vi "CommandServoPosition.vi"(7 "Debug with FS control?":bool, 8 "Error in":errorcluster, 9 "position [%FS]":dbl(slide) scale=-200.0..200.0, 10 "Suggested Rudder Setpoint":T1 min=-1.0 max=1.0 scale=1.0..-1.0, 11 "PWM Ref In":T2) -> (0 "Error out":errorcluster, 3 "duty cycle [%]":dbl)   [LabVIEW 2013]
doc: "This VI takes in a rudder setpoint in the RudderSuggestedSetpoint typedef (range of -1 to 1) and turns it into a a servo position. It is also passed a zero reference so that the rudder can be reinitialized to a new zero.\n\nAssumptions: there is a bound on the range of the rudder inside of this VI, set in consultation with the ME team. A zero position is also passed into this VI, which then translates an incoming -1 (full port) into the zero position minus half of the bounded range.\n\nThe 'Debug with FS Control?' boolean is made for TestRudderServo.vi, so the user can twiddle the servo around without any 'degrees to servo units' conversion. This should be used with new servos to get the 'degrees to servo units' conversion right.\n\nEric Schneider, March 2014"
uses:
  <vilib>/myRIO/Instrument Drivers/Onboard IO/PWM/typedefs/PWM Reference.ctl
  <vilib>/myRIO/Common/Instrument Driver Framework/Utilities/typedefs/myRIO Generic Hardware Reference.ctl
  <vilib>/myRIO/Common/Instrument Driver Framework/Utilities/typedefs/Hardware Version Enum.ctl
  <vilib>/myRIO/Common/Instrument Driver Framework/Utilities/typedefs/myRIO v1.0 Reference.ctl
  <vilib>/myRIO/Common/Instrument Driver Framework/Utilities/typedefs/Generic FPGA Reference.ctl
  <vilib>/myRIO/Common/Instrument Driver Framework/myRIO v1.0/PWM/typedefs/PWM Channels Enum.ctl
  <vilib>/myRIO/Instrument Drivers/Onboard IO/PWM/typedefs/PWM Configuration.ctl
  Data/TypeDefs/Rudder Set Suggestions.ctl
  <vilib>/Utility/error.llb/Error Cluster From Error Code.vi
  <vilib>/myRIO/Common/Instrument Driver Framework/myRIO v1.0/PWM/vis/myRIO v1.0 Write PWM.vi
  <vilib>/myRIO/Instrument Drivers/Onboard IO/PWM/PWM.lvlib
panel:
  in  "\"Zero\" reference (%FS units)":dbl format="%#_13g"
  in  "%FS per degree":dbl=1.85 format="%#_13g"
  in  "Desired range of rudder (deg)":dbl=60.0 format="%#_13g"
  out "offset [%FS]":dbl
  in  "null offset":bool
  out "pulse width [ms]":dbl=1.5
  in  "freq [Hz]":dbl=50.0
  # "Default settings from MyRIO example servo command code"
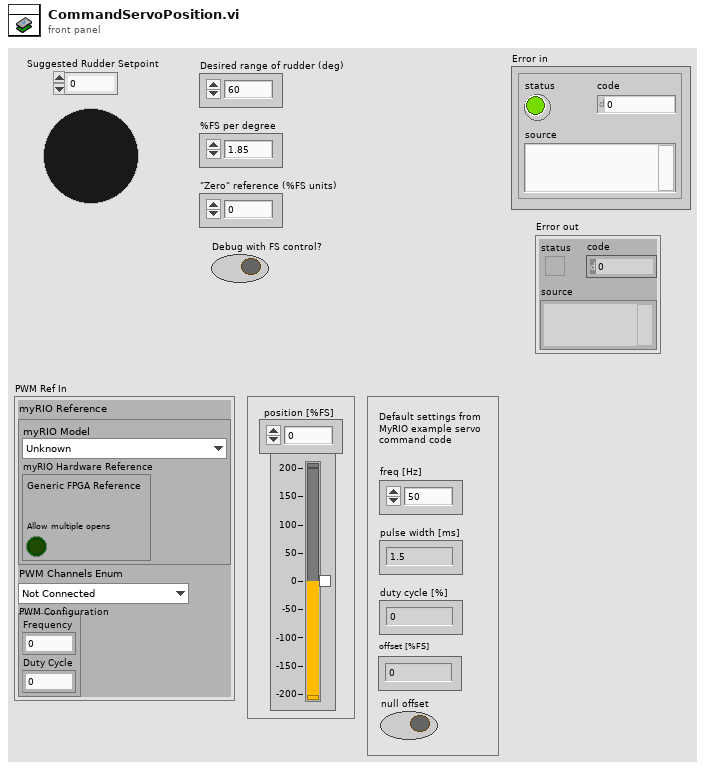
[diagram p1: front panel]
types:
  T1 = typedef "Rudder Set Suggestions.ctl" = dbl
  T2 = typedef "PWM.lvlib/PWM Reference.ctl" = cluster{"myRIO Reference":T3, "PWM Channels Enum":T7, "PWM Configuration":T8}
  T3 = typedef "myRIO Generic Hardware Reference.ctl" = cluster{"myRIO Model":T4, "myRIO Hardware Reference":T5}
  T4 = typedef "Hardware Version Enum.ctl" = enum16{"Unknown", "myRIO-1900", "myRIO-1950"}
  T5 = typedef "myRIO v1.0 Reference.ctl" = cluster{"Generic FPGA Reference":T6, "Allow multiple opens":bool}
  T6 = typedef "Generic FPGA Reference.ctl" = refnum<k20>
  T7 = typedef "PWM Channels Enum.ctl" = enum16{"Not Connected", "C/PWM0", "C/PWM1", "A/PWM0", "A/PWM1", "A/PWM2", "B/PWM0", "B/PWM1", "B/PWM2"}
  T8 = typedef "PWM.lvlib/PWM Configuration.ctl" = cluster{"Frequency":dbl, "Duty Cycle":dbl}
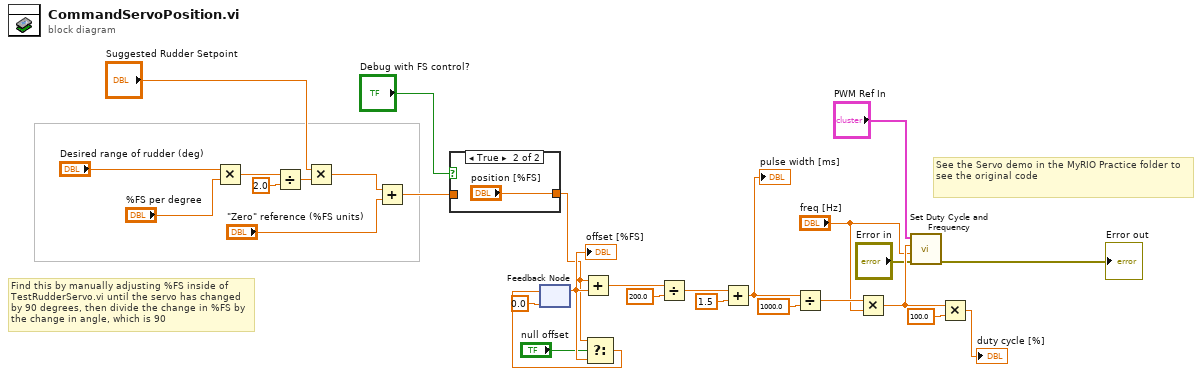
[diagram p0: block diagram]
diagram:
  # "Find this by manually adjusting %FS inside of TestRudderServo.vi until the servo has changed by 90 degrees, then divide the change in %FS by the change in angle, which is 90"
  # "See the Servo demo in the MyRIO Practice folder to see the original code"
  n1 = Multiply(x="Desired range of rudder (deg)", y="%FS per degree") -> (x*y=w8:dbl)
  n2 = Divide(x=w8, y=2.0) -> (x/y=w7:dbl)
  n3 = Multiply(x="Suggested Rudder Setpoint", y=w7) -> (x*y=w5:T1)
  n4 = Add(x=w5, y="\"Zero\" reference (%FS units)") -> (x+y=w2:T1)
  n5 = case shown="True" "Debug with FS control?" {
    tunnel: [w30 "position [%FS]"] -> w3
    tunnel: w2 -> [w30 _]
    frame False {
    }
    frame True {
    }
  }
  n6 = feedback #1(0.0 ("position [%FS]")) -> (w24:T1)
  "offset [%FS]" <- w24
  n7 = Add(x=w3, y=w24) -> (x+y=w23:T1)
  n8 = Select(t=w3, s="null offset", f=w24) -> (s? t:f=w22:T1)
  n9 = feedback-in #1(w22) -> ()
  n10 = Divide(x=w23, y=200.0) -> (x/y=w16:T1)
  n11 = Add(x=w16, y=1.5) -> (x+y=w18:T1)
  "pulse width [ms]" <- w18
  n12 = Divide(x=w18, y=1000.0) -> (x/y=w25:T1)
  n13 = Multiply(x=w25, y="freq [Hz]") -> (x*y=w28:T1)
  n14 = call <vilib>:"Set Duty Cycle and Frequency.vi"("error in (no error)"="Error in", "Frequency (Hz)"="freq [Hz]", "Duty Cycle (0-1)"=w28, "PWM Ref In"="PWM Ref In") -> ("error out"=→"Error out":errorcluster)  [unwired: 5 in, 1 out]
  n15 = Multiply(x=w28, y=100.0) -> (x*y=→"duty cycle [%]":T1)
